vi "Telemetry.vi"() -> ()   [LabVIEW 2012]
panel:
  in  "?":T1(tab)
  out "TCS":dbl
  out "LCS":dbl
  out "Numeric":dbl
  in  "MAPS":u16(ring) items=["POWER DRY", "POWER WET", "ECO DRY", "ECO WET", "ACCELERATION", "SKIDPAD"]
  out "GEAR":dbl
  out "LAMBDA":dbl
  out "P_SHIFT AIR TANK":dbl(knob) scale=0.0..10.0
  out "P_AIR 4":dbl(knob) scale=0.0..10.0
  out "P_CARTER":dbl(knob) scale=0.0..10.0
  out "P_FUEL":dbl(knob) scale=0.0..10.0
  out "P_OIL":dbl(knob) scale=0.0..10.0
  out "T_FUEL":dbl(slide) scale=0.0..100.0
  out "T_H20":dbl(slide) scale=0.0..100.0
  out "T_EXHAUST":dbl(slide) scale=0.0..100.0
  out "T_AIR":dbl(slide) scale=0.0..100.0
  out "T_OIL":dbl(slide) scale=0.0..100.0
  out "Throttle":u8(slide) scale=0.0..100.0
  out "RPM":dbl(knob) scale=13.0..13000.0
  out "Meter":dbl(knob) scale=-10.0..10.0
  out "Rear Brake":u8(slide) scale=0.0..100.0
  out "Throttle":u8(slide) scale=0.0..100.0
  out "Front Brake":u8(slide) scale=0.0..100.0
  out "?":dbl
  out "?":dbl
  out "?":dbl
  out "?":dbl
  out "?":dbl
  out "?":dbl
  out "?":dbl
  out "?":dbl
  out "Speed":dbl
  out "Gear":dbl
  in  "Chrono":i32(listbox)
  out "RPM":dbl(knob) scale=0.0..14.0
  out "?":u8(slide) scale=0.0..100.0
  out "?":dbl(slide) scale=0.0..250.0
  out "?":dbl(slide) scale=0.0..250.0
  out "?":u8(slide) scale=0.0..100.0
  in  "?":u32(colorbox)
  in  "?":u32(colorbox)
  in  "?":u32(colorbox)
  in  "?":u32(colorbox)
  in  "?":u32(colorbox)
  in  "?":u32(colorbox)
  out "?":u8(slide) scale=0.0..100.0
  out "?":dbl(slide) scale=0.0..250.0
  out "?":dbl(slide) scale=0.0..250.0
  out "?":u8(slide) scale=0.0..100.0
  in  "?":u32(colorbox)
  in  "?":u32(colorbox)
  in  "?":u32(colorbox)
  in  "?":u32(colorbox)
  in  "?":u32(colorbox)
  in  "?":u32(colorbox)
  out "Z ax":u8(slide) scale=0.0..100.0
  out "Rollio":cluster{dbl, dbl}(knob)={0.0, 6.215991901207513} scale=-10.0..10.0
  out "Tank":dbl(slide) scale=0.0..10.0
  out "Beccheggio":cluster{dbl, dbl}(knob)={0.0, -2.6548676720752784} scale=-10.0..10.0
  out "?":dbl(graph)
  out "XY ax":cluster{"Y":dbl[], "Y":dbl[]}[](graph)
  out "Waveform Chart 2":dbl(graph)
  # "PARTE MOTORE A REAL TIME"
  # "PARTE MOTORE PRE-PARTENZA (PRESO DALLA VECCHIA APP)"
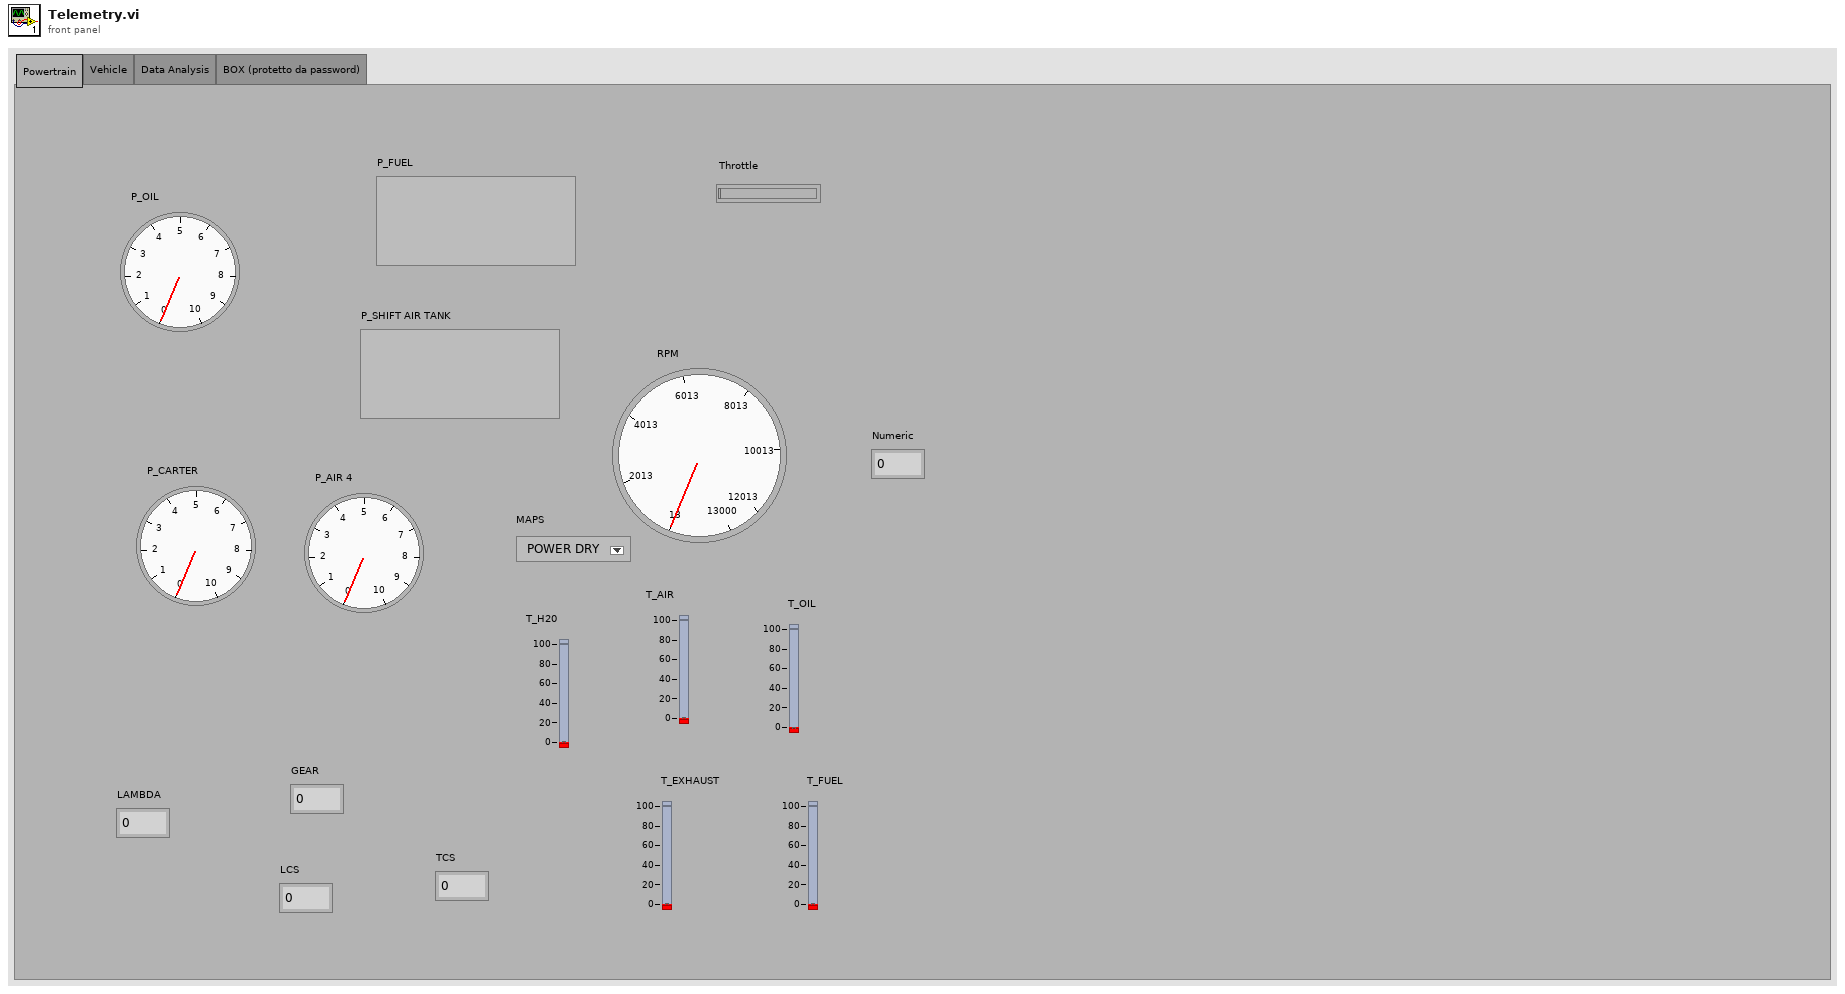
[diagram p1: front panel]
types:
  T1 = enum32{"Powertrain", "Vehicle", "Data Analysis", "BOX (protetto da password)"}
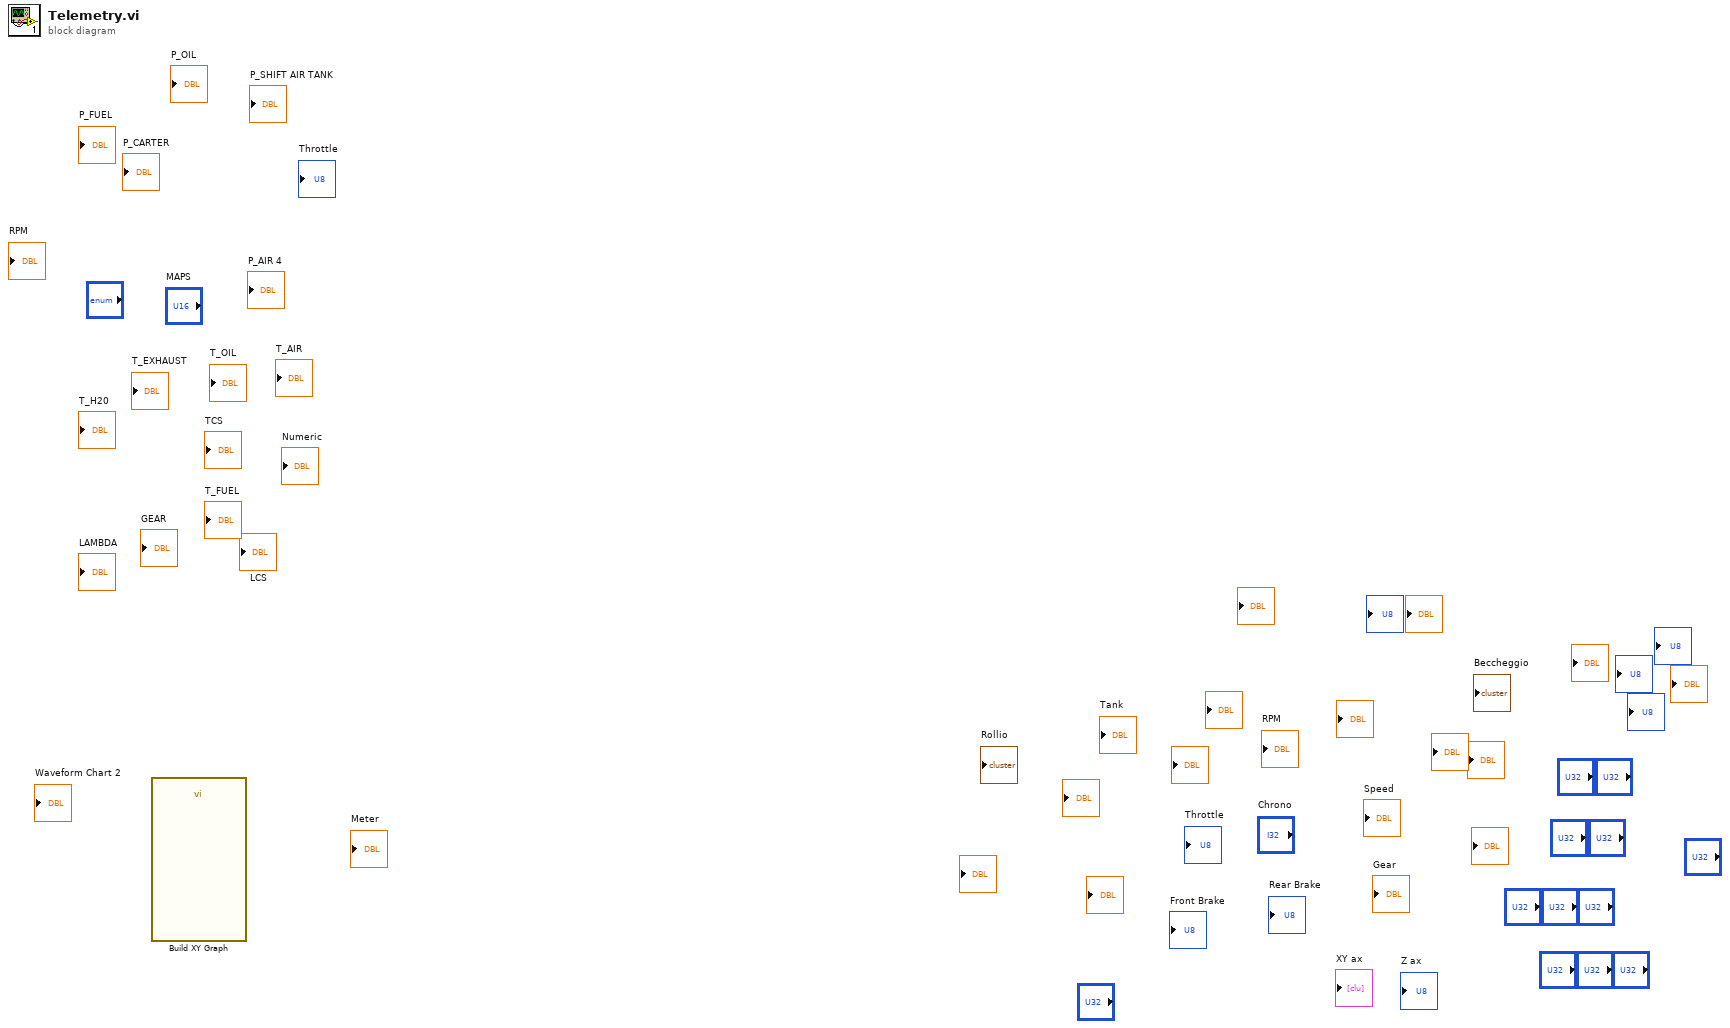
[diagram p0: block diagram]
diagram:
  n1 = call "Build XY Graph"() -> ()  [unwired: 5 in, 7 out]
